vi "Run.vi"(4 "Boolean":bool, 6 "Numeric":dbl, 7 "Database Entry in":refnum<class "Database Entry.lvclass">, 8 "error in (no error)":errorcluster, 9 "Assembly Type":string, 10 "Control In":T1={"I-O.lvclass"=refnum, "Gantry"=refnum, "Dispenser"="COM1"}, 11 "Assembly In":refnum<class "Calibrate.lvclass">) -> (0 "error out":errorcluster, 2 "Control Out":T1={"I-O.lvclass"=refnum, "Gantry"=refnum, "Dispenser"="COM1"}, 3 "Assembly Out":refnum<class "Calibrate.lvclass">, 5 "Database Entry out":refnum<class "Database Entry.lvclass">)   [LabVIEW 2021, in "Calibrate.lvclass"]
uses:
  Calibrate.lvclass
  Controller/Controllers.ctl
  Controller/I-O/I-O.lvclass
  C:/Program Files (x86)/Aerotech/A3200/LabVIEW/2010/Bin/Aerotech.A3200.dll
  Program Files (x86)/Aerotech/A3200/LabVIEW/2010/Bin/Aerotech.A3200.dll
  Database Entry/Database Entry.lvclass
  Calibrate.lvclass/Calibrate.ctl
  Assembly Run.lvclass
  Module/Module.lvclass
  Controller/Controller.lvclass
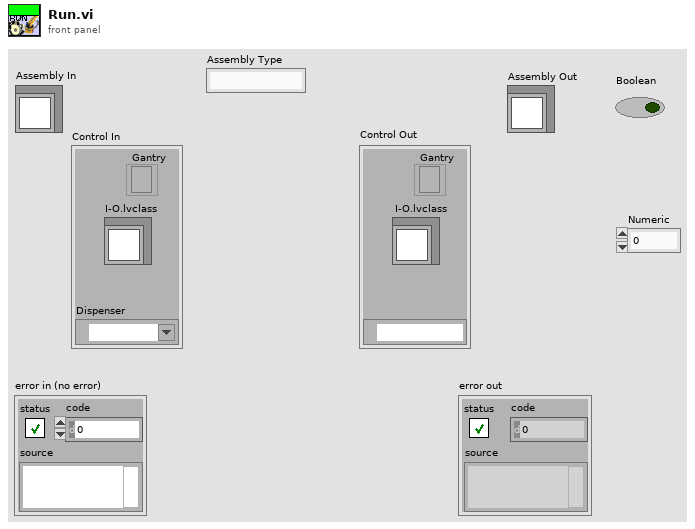
[diagram p1: front panel]
types:
  T1 = typedef "Controller.lvclass/Controllers.ctl" = cluster{"I-O.lvclass":refnum<class "I-O.lvclass">, "Gantry":refnum<k24>, "Dispenser":refnum<visa-resource-name>}
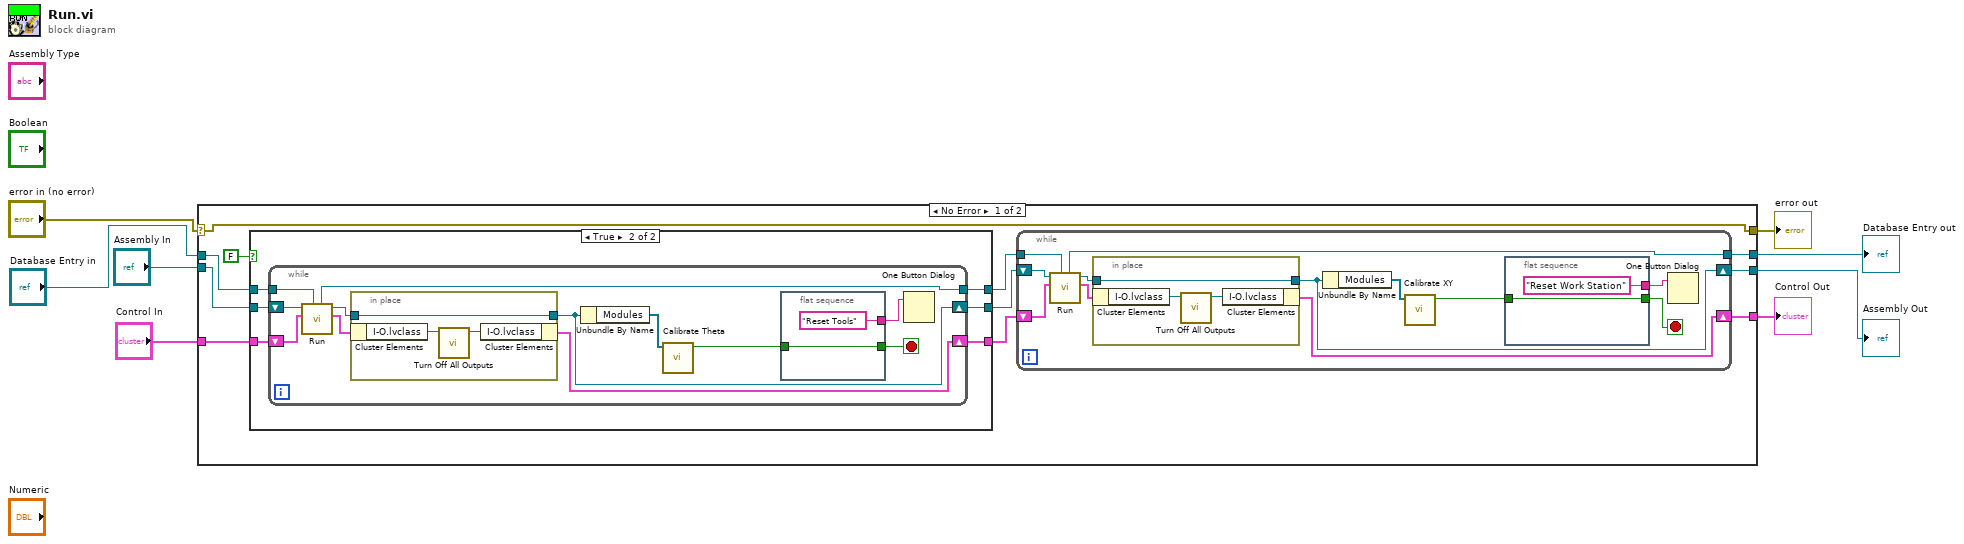
[diagram p0: block diagram]
diagram:
  n1 = case shown="No Error" "error in (no error)" {
    selector: "error in (no error)" -> [w13 w66]
    tunnel: "Control In" -> [w19 w64]
    tunnel: "Assembly In" -> [w17 w65]
    tunnel: [w16 w64] -> w6
    tunnel: [w14 w65] -> w5
    tunnel: [w13 w66] -> w3
    tunnel: "Database Entry in" -> [w10 w63]
    tunnel: [w11 w63] -> w1
    frame No Error {
      n2 = case shown="True" FALSE {
        tunnel: w19 -> [w21 w28]
        tunnel: [w21 w27] -> w18
        tunnel: w17 -> [w22 w26]
        tunnel: [w22 w25] -> w15
        tunnel: w10 -> [w20 w24]
        tunnel: [w20 w23] -> w9
        frame False {
        }
        frame True {
          n3 = while {
            shift-right: [w34] -> w27
            shift-left: w28 -> [w40]
            shift-right: [w31] -> w25
            shift-left: w26 -> [w39]
            tunnel: w24 -> [w30]
            tunnel: [w29] -> w23
            stop <- w32 stop-if-true
            n4 = call-parent "Run.vi"("Database Entry in"=w30, "Control In"=w40, "Assembly In"=w39) -> ("Control Out"=w36:T1, "Assembly Out"=w35:refnum<class "Calibrate.lvclass">, "Database Entry out"=w29:refnum<class "Database Entry.lvclass">)  [unwired: 5 in, 1 out]
            n5 = in-place {
              in-place-border: w35 -> [w41]
              in-place-border: [w41] -> w31
              n6 = in-place-cluster #1(w36) -> ("I-O.lvclass"=w43:refnum<class "I-O.lvclass">)
              n7 = call-dynamic "Turn Off All Outputs.vi"("I-O in"=w43) -> ("I-O out"=w42:refnum<class "I-O.lvclass">)  [unwired: 9 in, 1 out]
              n8 = in-place-cluster #1("I-O.lvclass"=w42) -> (w34:T1)
            }
            n9 = Unbundle By Name(w31) -> ("Modules"=w38:refnum<class "Module.lvclass">[])
            n10 = call "Calibrate Theta.vi"("Modules"=w38) -> ("Continue?"=w33:bool)  [unwired: 10 in]
            n11 = flat-sequence {
              tunnel: ["Reset Tools"] -> w37
              tunnel: w33 -> [w44]
              tunnel: [w44] -> w32
              frame #0 {
              }
            }
            n12 = One Button Dialog(message=w37) -> ()  [unwired: 1 in, 1 out]
          }
        }
      }
      n13 = while {
        shift-right: [w48] -> w16
        shift-left: w18 -> [w56]
        shift-right: [w49] -> w14
        shift-left: w15 -> [w57]
        tunnel: w9 -> [w47]
        tunnel: [w46] -> w11
        stop <- w52 stop-if-true
        n14 = call-parent "Run.vi"("Database Entry in"=w47, "Control In"=w56, "Assembly In"=w57) -> ("Control Out"=w51:T1, "Assembly Out"=w50:refnum<class "Calibrate.lvclass">, "Database Entry out"=w46:refnum<class "Database Entry.lvclass">)  [unwired: 5 in, 1 out]
        n15 = in-place {
          in-place-border: w50 -> [w58]
          in-place-border: [w58] -> w49
          n16 = in-place-cluster #2(w51) -> ("I-O.lvclass"=w60:refnum<class "I-O.lvclass">)
          n17 = call-dynamic "Turn Off All Outputs.vi"("I-O in"=w60) -> ("I-O out"=w59:refnum<class "I-O.lvclass">)  [unwired: 9 in, 1 out]
          n18 = in-place-cluster #2("I-O.lvclass"=w59) -> (w48:T1)
        }
        n19 = Unbundle By Name(w49) -> ("Modules"=w55:refnum<class "Module.lvclass">[])
        n20 = call "Calibrate XY.vi"("Modules"=w55) -> ("Continue?"=w53:bool)  [unwired: 10 in]
        n21 = flat-sequence {
          tunnel: ["Reset Work Station"] -> w54
          tunnel: w53 -> [w61]
          tunnel: [w61] -> w52
          frame #0 {
          }
        }
        n22 = One Button Dialog(message=w54) -> ()  [unwired: 1 in, 1 out]
      }
    }
    frame Error {
    }
  }
  "error out" <- w3
  "Control Out" <- w6
  "Assembly Out" <- w5
  "Database Entry out" <- w1
